vi "Create.vi"(7 "x":dbl, 8 "error in":errorcluster, 9 "w":dbl, 10 "z":dbl, 11 "y":dbl) -> (0 "error out":errorcluster, 3 "Orient3d out":refnum<class "Orient3d Class.lvclass">)   [LabVIEW 2011, in "Orient3d Class.lvclass"]
uses:
  Orient3d Class.lvclass
  Orient3d Class.lvclass/Orient3d Class.ctl
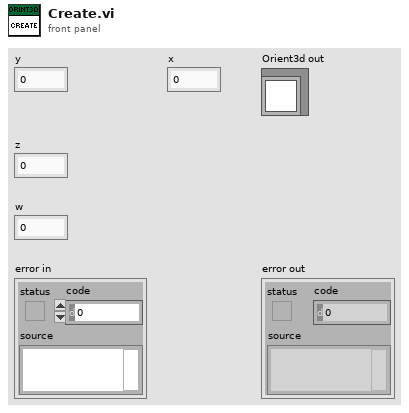
[diagram p1: front panel]
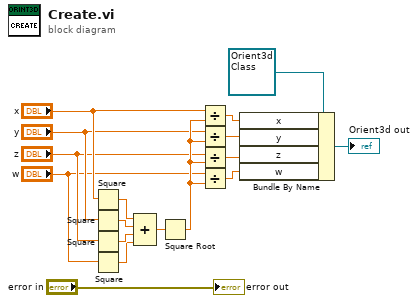
[diagram p0: block diagram]
diagram:
  n1 = Square(x="x") -> (x^2=w13:dbl)
  n2 = Square(x="y") -> (x^2=w14:dbl)
  n3 = Square(x="z") -> (x^2=w12:dbl)
  n4 = Square(x="w") -> (x^2=w11:dbl)
  n5 = Compound Arithmetic op=ADD(w13, w14, w12, w11) -> (w10:dbl)
  n6 = Square Root(x=w10) -> (sqrt(x)=w5:dbl)
  n7 = Divide(x="x", y=w5) -> (x/y=w9:dbl)
  n8 = Divide(x="y", y=w5) -> (x/y=w8:dbl)
  n9 = Divide(x="z", y=w5) -> (x/y=w7:dbl)
  n10 = Divide(x="w", y=w5) -> (x/y=w6:dbl)
  n11 = Bundle By Name(cluster=refnum<class "Orient3d Class.lvclass"> refnum ("Orient3d Class in"), "x"=w9, "y"=w8, "z"=w7, "w"=w6) -> (→"Orient3d out":refnum<class "Orient3d Class.lvclass">)
  "error out" <- "error in"
